vi "Data cumulation(DBL).vi"(8 "error in (no error)":errorcluster, 10 "Data in":dbl format="%#_13g", 11 "Sample length":i32) -> (0 "error out":errorcluster, 1 "Data out":dbl[](array[numeric]), 2 "Counter":i32, 3 "Data status":enum16{"Data not ready", "Data ready"}(ring))   [LabVIEW 2013]
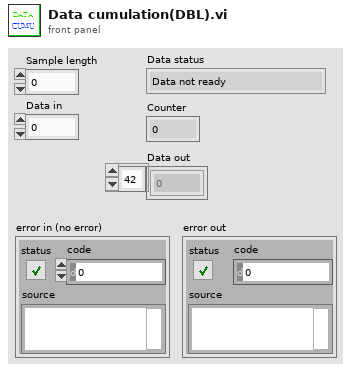
[diagram p1: front panel]
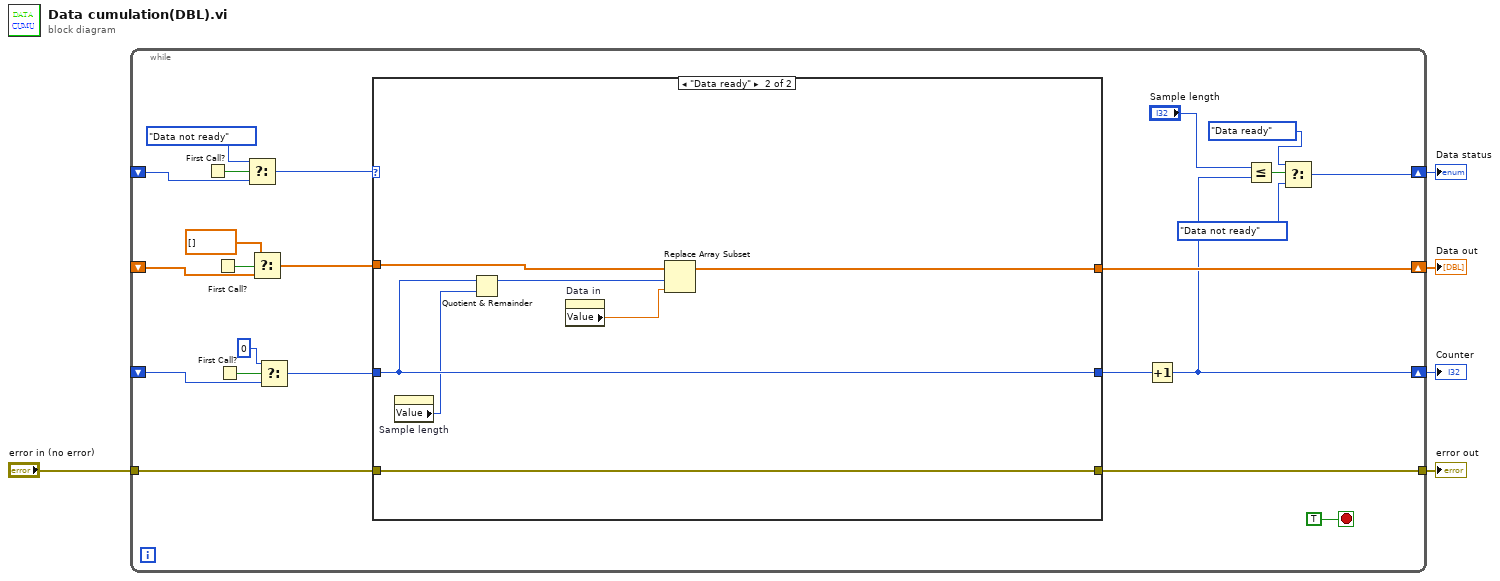
[diagram p0: block diagram]
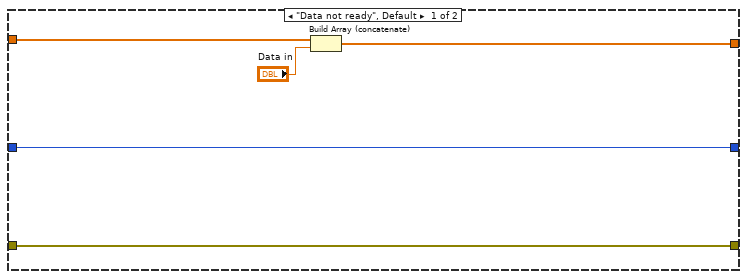
[diagram p2: hidden frame]
diagram:
  n1 = while {
    shift-right: [w18] -> w4
    shift-left: _ -> [w8]
    shift-right: [w23] -> w5
    shift-left: _ -> [w21]
    shift-right: [w12] -> w3
    shift-left: _ -> [w15]
    tunnel: "error in (no error)" -> [w11]
    tunnel: [w10] -> w1
    stop <- TRUE stop-if-true
    n2 = First Call?() -> (First Call?: T/F=w22:bool)
    n3 = First Call?() -> (First Call?: T/F=w9:bool)
    n4 = First Call?() -> (First Call?: T/F=w17:bool)
    n5 = Select(t=enum16{"Data not ready", "Data ready"}."Data not ready", s=w22, f=w21) -> (s? t:f=w19:enum16{"Data not ready", "Data ready"})
    n6 = Select(t=dbl[] [], s=w9, f=w8) -> (s? t:f=w6:dbl[])
    n7 = Select(t=0, s=w17, f=w15) -> (s? t:f=w14:i32)
    n8 = case shown="\"Data ready\"" w19 {
      tunnel: w6 -> [w32 w39]
      tunnel: [w31 w35] -> w18
      tunnel: w14 -> [w30 w37]
      tunnel: [w30 w37] -> w13
      tunnel: w11 -> [w29 w34]
      tunnel: [w29 w34] -> w10
      frame "Data not ready", Default {
        n9 = Build Array (concatenate)(w32, "Data in") -> (w31:dbl[])
      }
      frame "Data ready" {
        n10 = property on="Sample length" class="DigNum (strict)"() -> ("Value"=w36:i32)  [unwired: 2 in, 2 out]
        n11 = Quotient & Remainder(x=w37, y=w36) -> (x-y*floor(x/y)=w40:i32)  [unwired: 1 out]
        n12 = property on="Data in" class="DigNum (strict)"() -> ("Value"=w38:dbl)  [unwired: 2 in, 2 out]
        n13 = Replace Array Subset(array=w39, new element=w38, index=w40) -> (w35:dbl[])
      }
    }
    n14 = Increment(x=w13) -> (x+1=w12:i32)
    n15 = Less Or Equal?(x="Sample length", y=w12) -> (x <= y?=w26:bool)
    n16 = Select(t=enum16{"Data not ready", "Data ready"}."Data ready", s=w26, f=enum16{"Data not ready", "Data ready"}."Data not ready") -> (s? t:f=w23:enum16{"Data not ready", "Data ready"})
  }
  "Data status" <- w5
  "Data out" <- w4
  "Counter" <- w3
  "error out" <- w1
